vi "setReferenceOscillator.vi"(8 "error in (no error)":errorcluster, 10 "Mode":enum16{"Internal", "External", "Auto"}(ring), 11 "VISA resource name":refnum<visa-resource-name>) -> (0 "error out":errorcluster, 3 "VISA resource name out":refnum<visa-resource-name>)   [LabVIEW 2023, in "Keysight-33500B.lvlib"]
doc: "<b>Author:</b> Wolfgang\n<b>Description:</b>\nThe ROSCillator subsystem controls use of the 10 MHz reference oscillator and external reference\noscillator input. The reference oscillator is the primary clock for all waveform synthesis. All waveforms are\nphase-locked to the reference oscillator, which therefore controls output signal frequency and phase."
uses:
  Keysight-33500B.lvlib
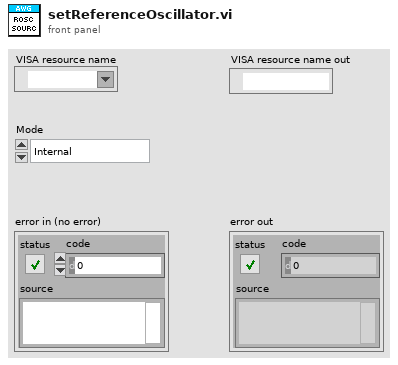
[diagram p1: front panel]
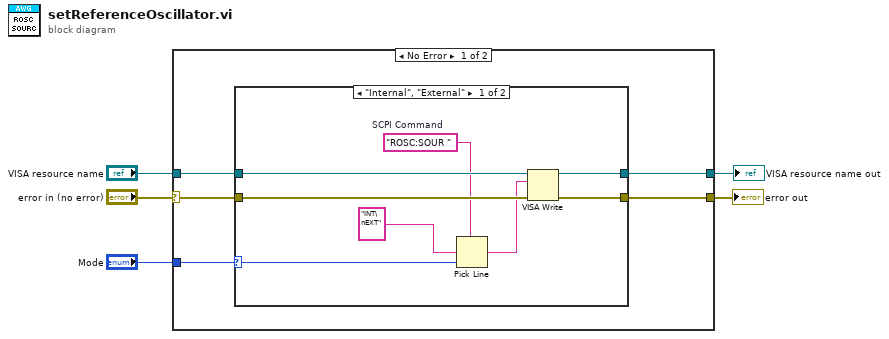
[diagram p0: block diagram]
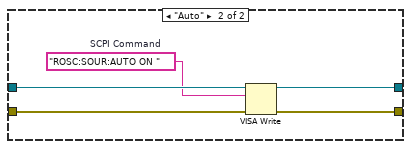
[diagram p2: hidden frame]
diagram:
  n1 = case shown="No Error" "error in (no error)" {
    selector: "error in (no error)" -> [w7 w25]
    tunnel: [w9 w24] -> w5
    tunnel: [w10 w25] -> w3
    tunnel: "VISA resource name" -> [w8 w24]
    tunnel: "Mode" -> [w6 _]
    frame No Error {
      n2 = case shown="\"Internal\", \"External\"" w6 {
        selector: w6 -> [w14 _]
        tunnel: [w18 w23] -> w10
        tunnel: [w17 w22] -> w9
        tunnel: w8 -> [w16 w21]
        tunnel: w7 -> [w15 w20]
        frame "Internal", "External" {
          w13 = "ROSC:SOUR "  # SCPI Command
          n3 = Pick Line(string ("")=w13, multi-line string="INT\nEXT", line index=w14) -> (output string=w12:string)
          n4 = VISA Write(VISA resource name=w16, write buffer=w12, error in (no error)=w15) -> (VISA resource name out=w17:refnum<visa-resource-name>, error out=w18:errorcluster)  [unwired: 1 out]
        }
        frame "Auto" {
          w19 = "ROSC:SOUR:AUTO ON "  # SCPI Command
          n5 = VISA Write(VISA resource name=w21, write buffer=w19, error in (no error)=w20) -> (VISA resource name out=w22:refnum<visa-resource-name>, error out=w23:errorcluster)  [unwired: 1 out]
        }
      }
    }
    frame Error {
    }
  }
  "VISA resource name out" <- w5
  "error out" <- w3
